vi "QD Clear Debug Snapshot.vi"(6 "Variant in":variant, 7 "Shift Pressed?":bool, 8 "error in (no error)":errorcluster, 10 "QD Combo Box Ref":refnum<vi>, 11 "QD Launch VI Ref":refnum<vi>) -> (0 "error out":errorcluster, 4 "Variant out":variant)   [LabVIEW 2020]
doc: "Clears stored <b>Debug Snapshot</b> for the active VI. Use SHIFT to delete the cache file.\n\nDefault Shortcut - [c]"
uses:
  Public API.lvlib
  Path Getter/Path Getter.lvclass
  C:/Users/juanj/Documents/hasbun_wood_engineering/github/Debug-Snapshots-for-LabVIEW/src/Path Getter/Path Getter.lvclass
  C:/Users/juanj/Documents/hasbun_wood_engineering/github/Debug-Snapshots-for-LabVIEW/src/IPath Getter/IPath Getter.lvclass
panel:
  in  "Undo Name":string="Quick Drop Keyboard Shortcut"
  # "Do not change the connector pane of this VI.\n\nSee the block diagram for directions on how to use this template."
  # "Specify the name of the Undo transaction"
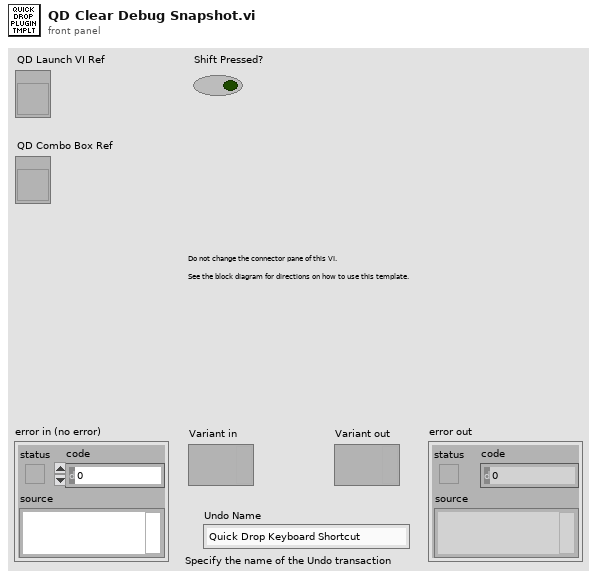
[diagram p1: front panel]
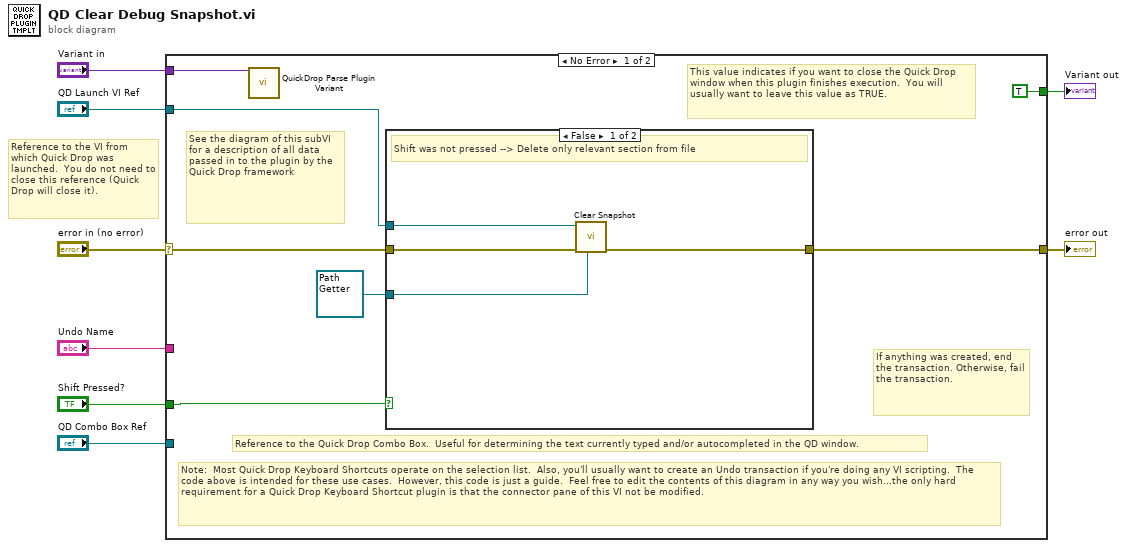
[diagram p0: block diagram]
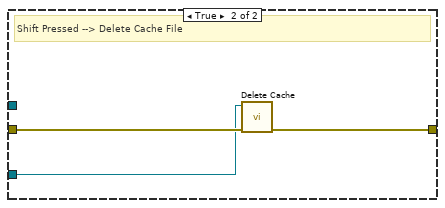
[diagram p2: hidden frame]
diagram:
  # "Reference to the VI from which Quick Drop was launched.  You do not need to close this reference (Quick Drop will close it)."
  n1 = case shown="No Error" "error in (no error)" {
    selector: "error in (no error)" -> [w13 w23]
    tunnel: [w11 w23] -> w7
    tunnel: "QD Launch VI Ref" -> [w10 _]
    tunnel: "Shift Pressed?" -> [w12 _]
    tunnel: "QD Combo Box Ref" -> [_ _]
    tunnel: "Variant in" -> [w15 _]
    tunnel: "Undo Name" -> [_ _]
    tunnel: [TRUE _] -> w1
    frame No Error {
      # "Note:  Most Quick Drop Keyboard Shortcuts operate on the selection list.  Also, you'll usually want to create an Undo transaction if you're doing any VI scripting.  The code above is intended for these use cases.  However, this code is just a guide.  Feel free to edit the contents of this diagram in any way you wish...the only hard requirement for a Quick Drop Keyboard Shortcut plugin is that the connector pane of this VI not be modified."
      # "If anything was created, end the transaction. Otherwise, fail the transaction."
      # "This value indicates if you want to close the Quick Drop window when this plugin finishes execution.  You will usually want to leave this value as TRUE."
      # "See the diagram of this subVI for a description of all data passed in to the plugin by the Quick Drop framework"
      # "Reference to the Quick Drop Combo Box.  Useful for determining the text currently typed and/or autocompleted in the QD window."
      n2 = call <vilib>:"QuickDrop Parse Plugin Variant.vi"("QDKS Variant in"=w15) -> ()  [unwired: 12 in, 3 out]
      n3 = case shown="False" w12 {
        tunnel: w13 -> [w19 w22]
        tunnel: [w18 w21] -> w11
        tunnel: w10 -> [w17 _]
        tunnel: refnum<class "Path Getter.lvclass"> refnum ("Path Getter.lvclass") -> [w16 w20]
        frame False {
          # "Shift was not pressed --> Delete only relevant section from file"
          n4 = call "Clear Snapshot.vi"("IPath Getter.lvclass"=w16, "error in"=w19, "VI Reference in"=w17) -> ("error out"=w18:errorcluster)  [unwired: 7 in, 1 out]
        }
        frame True {
          # "Shift Pressed --> Delete Cache File"
          n5 = call "Delete Cache.vi"("error in"=w22, "IPath Getter.lvclass"=w20) -> ("error out"=w21:errorcluster)  [unwired: 9 in]
        }
      }
    }
    frame Error {
    }
  }
  "error out" <- w7
  "Variant out" <- w1
